vi "Get Variables.vi"(8 "error in (no error)":errorcluster, 11 "Comparison Operations in":refnum<class "Comparison Functions.lvclass">) -> (0 "error out":errorcluster, 2 "Variables":variant, 3 "Comparison Operations out":refnum<class "Comparison Functions.lvclass">)   [LabVIEW 2019, in "Comparison Functions.lvclass"]
uses:
  Comparison Functions.lvclass
  Comparison Functions.lvclass/Comparison Functions.ctl
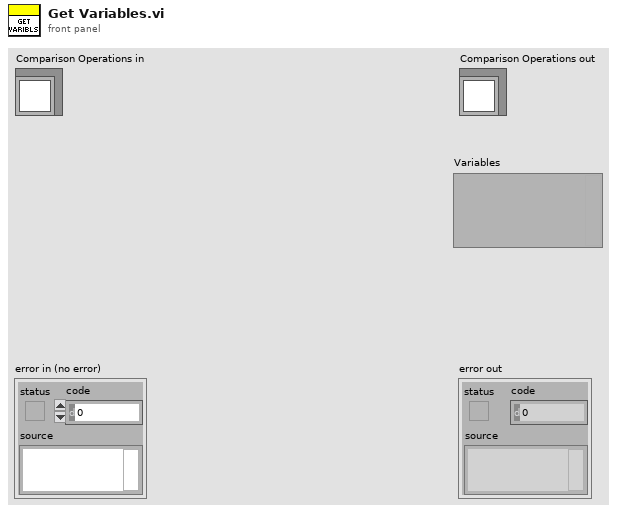
[diagram p1: front panel]
types:
  T1 = typedef "Comparison Functions.lvclass/Variables.ctl" = cluster{"Var1":variant, "Var2":variant}
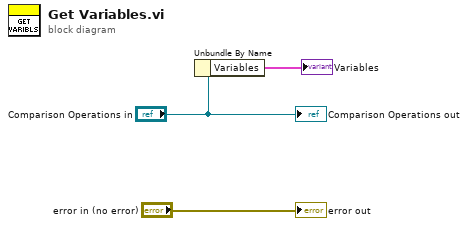
[diagram p0: block diagram]
diagram:
  n1 = Unbundle By Name("Comparison Operations in") -> ("Variables"=→"Variables":T1)
  "error out" <- "error in (no error)"
  "Comparison Operations out" <- "Comparison Operations in"
